vi "experienceNetworkLatency.vi"(8 "error in (no error)":errorcluster) -> (0 "error out":errorcluster)   [LabVIEW 2017, in "ThirdPartyYoutubeClass.lvclass"]
uses:
  ThirdPartyYoutubeClass.lvclass
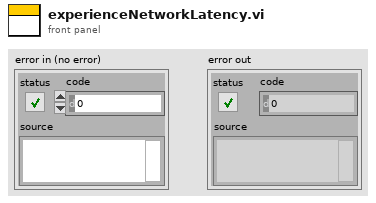
[diagram p1: front panel]
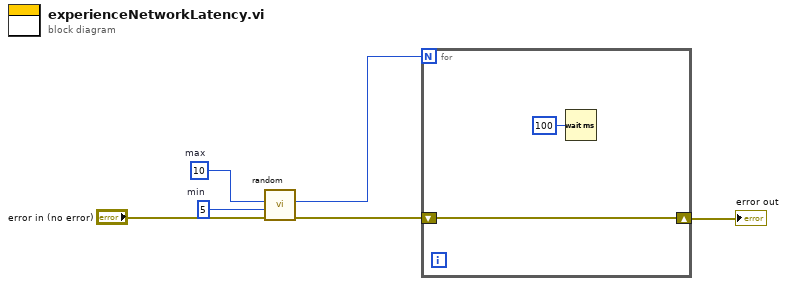
[diagram p0: block diagram]
diagram:
  w2 = 10  # max
  w3 = 5  # min
  n1 = call "random.vi"("error in (no error)"="error in (no error)", "min"=w3, "max"=w2) -> ("error out"=w4:errorcluster, "random"=w1:i32)  [unwired: 7 in]
  n2 = for {
    N: w1 -> [_]
    shift-right: [w8] -> w5
    shift-left: w4 -> [w8]
    n3 = Wait (ms)(milliseconds to wait=u32 100) -> ()  [unwired: 1 out]
  }
  "error out" <- w5
